vi "Configure Flowrate.vi"(8 "error in (no error)":errorcluster, 10 "Flowrate (1 ml/min)":dbl, 11 "VISA resource name":refnum<visa-resource-name>) -> (0 "error out":errorcluster, 3 "VISA resource name out":refnum<visa-resource-name>)   [LabVIEW 2018]
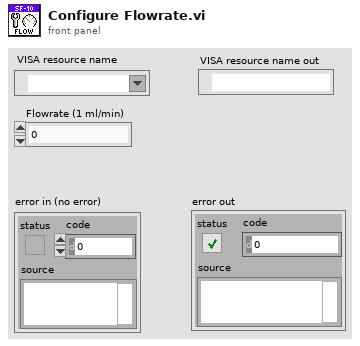
[diagram p1: front panel]
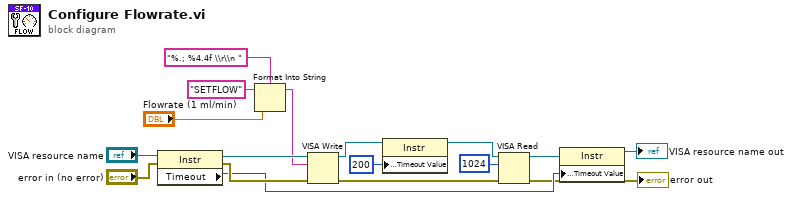
[diagram p0: block diagram]
diagram:
  n1 = property class="Instr"(reference="VISA resource name", error in="error in (no error)") -> (reference out=w15:refnum<visa-resource-name>, error out=w14:errorcluster, "Timeout"=w10:u32)
  n2 = Format Into String(format string="%.; %4.4f \\r\\n ", initial string="SETFLOW", "Flowrate (1 ml/min)") -> (resulting string=w6:string)  [unwired: 1 in, 1 out]
  n3 = VISA Write(VISA resource name=w15, write buffer=w6, error in (no error)=w14) -> (VISA resource name out=w2:refnum<visa-resource-name>, error out=w9:errorcluster)  [unwired: 1 out]
  n4 = property class="Instr"(reference=w2, "General Settings:Timeout Value"=u32 200) -> (reference out=w1:refnum<visa-resource-name>)  [unwired: 1 in, 1 out]
  n5 = VISA Read(VISA resource name=w1, byte count=u32 1024, error in (no error)=w9) -> (VISA resource name out=w11:refnum<visa-resource-name>, error out=→"error out":errorcluster)  [unwired: 2 out]
  n6 = property class="Instr"(reference=w11, "General Settings:Timeout Value"=w10) -> (reference out=→"VISA resource name out":refnum<visa-resource-name>)  [unwired: 1 in, 1 out]
